vi "Post Message.vi"(8 "Error in":errorcluster caption="Error in (no error)", 9 "Module Name":string, 10 "Argument(\"\")":string, 11 "Message":string) -> (0 "Error out":errorcluster)   [LabVIEW 2017, in "_csmlite.lvlib"]
uses:
  _csmlite.lvlib
  _action.ctl
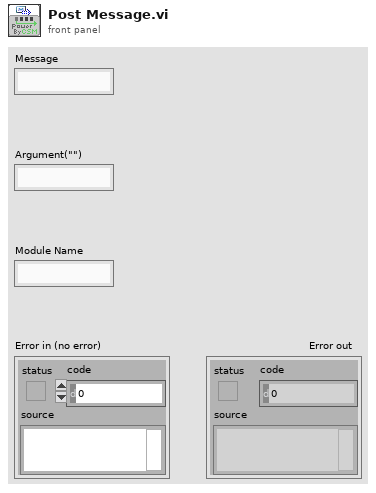
[diagram p1: front panel]
types:
  T1 = typedef "_csmlite.lvlib/_action.ctl" = enum16{"Obtain", "Destroy", "Broadcast", "Post"}
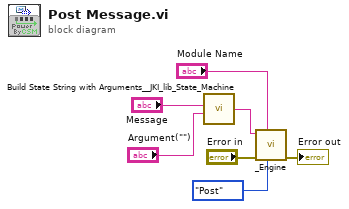
[diagram p0: block diagram]
diagram:
  n1 = call <vilib>:"Build State String with Arguments__JKI_lib_State_Machine.vi"("Arguments (\"\")"="Argument(\"\")", "State"="Message") -> ("State with Arguments"=w4:string)  [unwired: 4 in]
  n2 = call "_Engine.vi"("Enum"=_action."Post", "Module Name"="Module Name", "Error in"="Error in", "Message"=w4) -> ("Error out"=→"Error out":errorcluster)  [unwired: 6 in, 1 out]
